vi "SimpleSerialTest.vi"() -> ()   [LabVIEW 2013]
uses:
  Data/TypeDefs/Notifiers.ctl
  Data/TypeDefs/UTM Location.ctl
  Data/TypeDefs/Sail Set Suggestions.ctl
  Data/TypeDefs/Rudder Set Suggestions.ctl
  Data/TypeDefs/OverrideInformation.ctl
  Data/TypeDefs/OverrideMode.ctl
  Data/TypeDefs/MotorSetup.ctl
  Data/TypeDefs/DynamixelSetupInfo.ctl
  Data/TypeDefs/AirmarStatus.ctl
  Data/TypeDefs/HardwareOnline.ctl
  Data/TypeDefs/DynamixelCycleTracker.ctl
  Data/TypeDefs/RC Input Values.ctl
  Classes/Waypoint/Waypoint.lvclass
  Data/TypeDefs/GPS-Compass Queue Cluster.ctl
  Data/TypeDefs/WindData Queue Cluster.ctl
  <vilib>/Instr/_visa.llb/VISA Configure Serial Port (Instr).vi
panel:
  out "Loop Frequency":dbl(graph)
  out "Loop Frequency (Hz)":dbl
  in  "Cycles per buffer flush":i32=1000
  out "Sentence":string
  in  "stop":bool
  out "While counter":i32
  in  "NotifierReff":T1
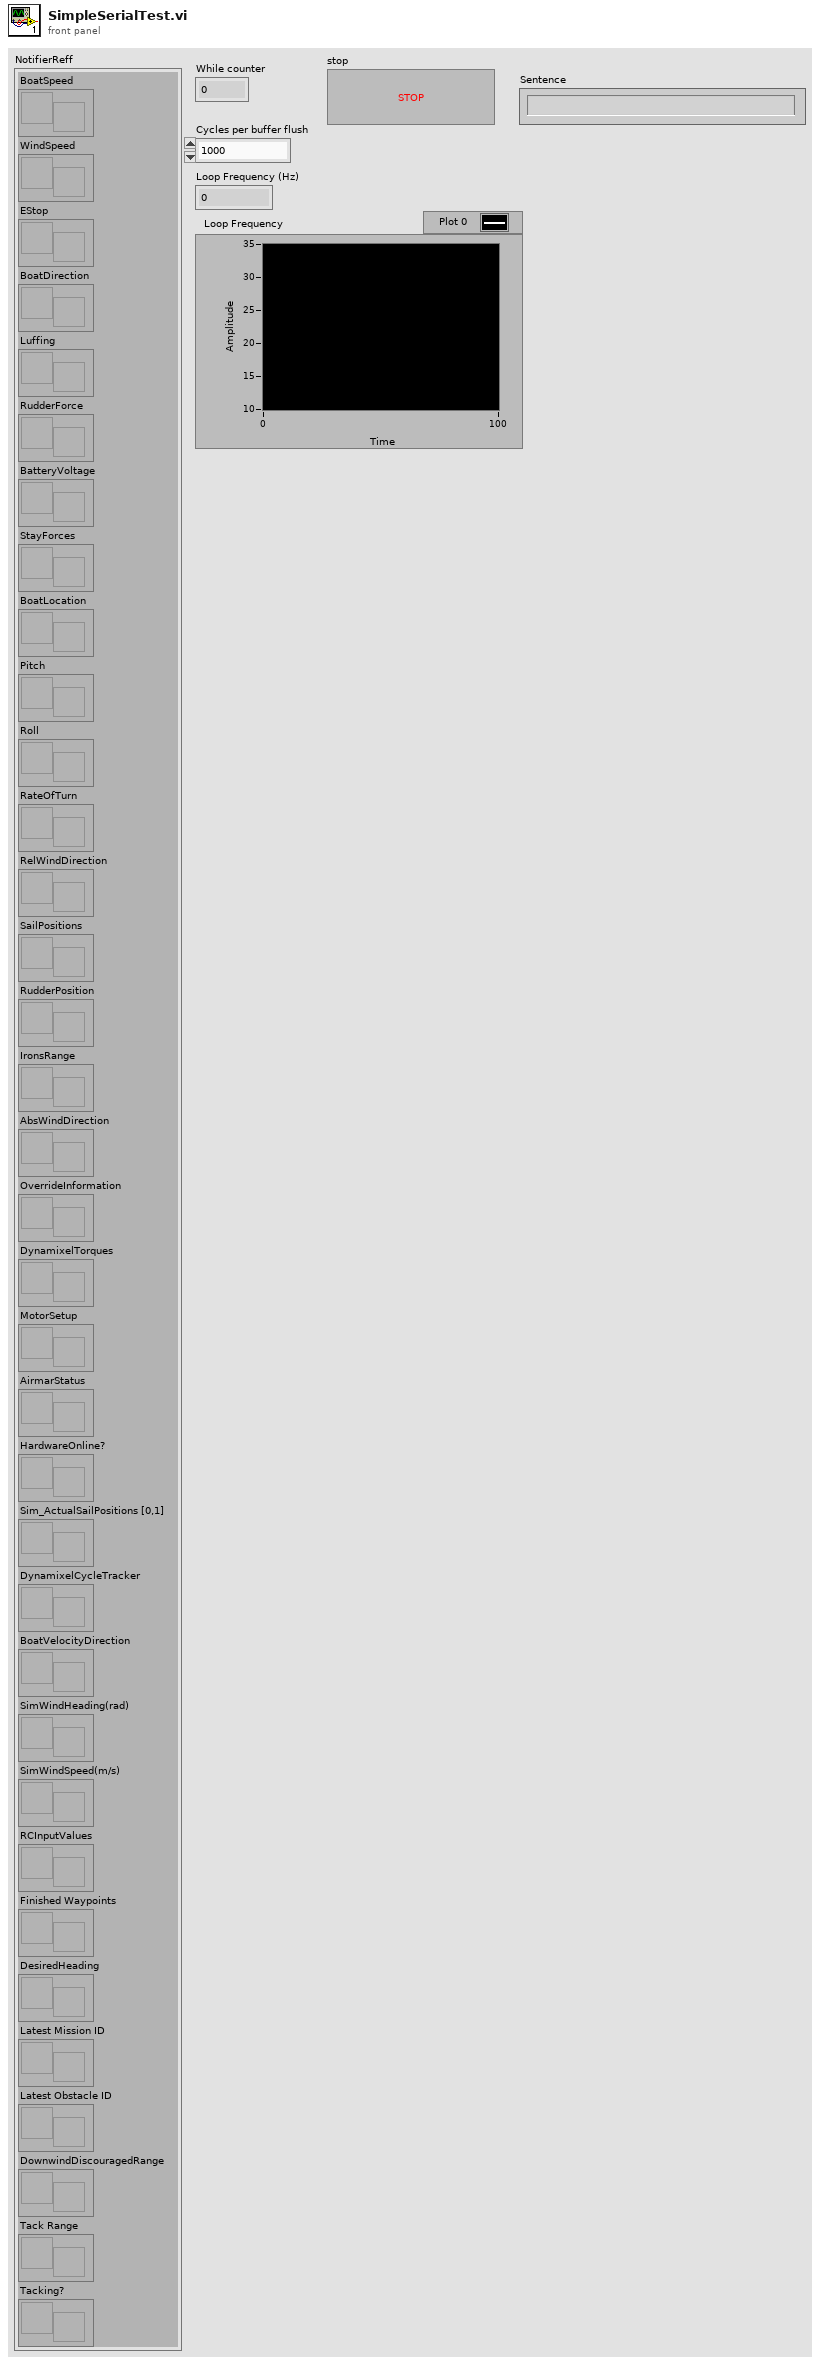
[diagram p1: front panel]
types:
  T1 = typedef "Notifiers.ctl" = cluster{"BoatSpeed":refnum<notifier>, "WindSpeed":refnum<notifier>, "EStop":refnum<notifier>, "BoatDirection":refnum<notifier>, "Luffing":refnum<notifier>, "RudderForce":refnum<notifier>, "BatteryVoltage":refnum<notifier>, "StayForces":refnum<notifier>, "BoatLocation":refnum<notifier>, "Pitch":refnum<notifier>, "Roll":refnum<notifier>, "RateOfTurn":refnum<notifier>, "RelWindDirection":refnum<notifier>, "SailPositions":refnum<notifier>, "RudderPosition":refnum<notifier>, "IronsRange":refnum<notifier>, "AbsWindDirection":refnum<notifier>, "OverrideInformation":refnum<notifier>, "DynamixelTorques":refnum<notifier>, "MotorSetup":refnum<notifier>, "AirmarStatus":refnum<notifier>, "HardwareOnline?":refnum<notifier>, "Sim_ActualSailPositions [0,1]":refnum<notifier>, "DynamixelCycleTracker":refnum<notifier>, "BoatVelocityDirection":refnum<notifier>, "SimWindHeading(rad)":refnum<notifier>, "SimWindSpeed(m/s)":refnum<notifier>, "RCInputValues":refnum<notifier>, "Finished Waypoints":refnum<notifier>, "DesiredHeading":refnum<notifier>, "Latest Mission ID":refnum<notifier>, "Latest Obstacle ID":refnum<notifier>, "DownwindDiscouragedRange":refnum<notifier>, "Tack Range":refnum<notifier>, "Tacking?":refnum<notifier>}
  T2 = typedef "WindData Queue Cluster.ctl" = cluster{"RelWindDirection Queue":refnum<queue>, "WindSpeed Queue":refnum<queue>, "AbsWindDirection Queue":refnum<queue>}
  T3 = typedef "GPS-Compass Queue Cluster.ctl" = cluster{"BoatLocation Queue":refnum<queue>, "BoatDirection Queue":refnum<queue>, "BoatSpeed Queue":refnum<queue>, "RateOfTurn Queue":refnum<queue>, "Pitch Queue":refnum<queue>, "Roll Queue":refnum<queue>, "BoatVelocityDirection Queue ":refnum<queue>}
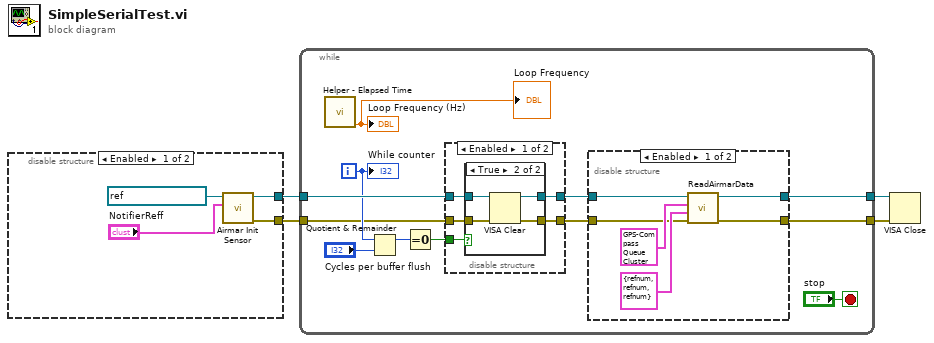
[diagram p0: block diagram]
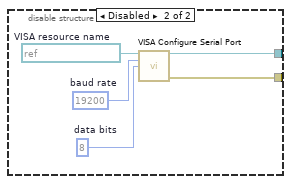
[diagram p2: hidden frame]
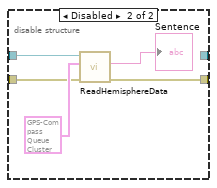
[diagram p5: hidden frame]
diagram:
  n1 = disable-structure shown="Enabled" {
    disable-tunnel: [w6 w10] -> w4
    disable-tunnel: [w5 w9] -> w2
    frame Enabled {
      n2 = call "Airmar Init Sensor.vi"("NotifierReff"="NotifierReff", "VISA Refnum in"=refnum<visa-resource-name> "ASRL2::INSTR") -> ("error out"=w5:errorcluster, "VISA Refnum out"=w6:refnum<visa-resource-name>)  [unwired: 7 in, 1 out]
    }
    frame Disabled {
      w13 = u16 8  # data bits
      w11 = u32 19200  # baud rate
      w12 = refnum<visa-resource-name> "ASRL2::INSTR"  # VISA resource name
      n3 = call-poly "VISA Configure Serial Port"("VISA resource name"=w12, "baud rate (9600)"=w11, "data bits (8)"=w13) -> ("VISA resource name out"=w10:refnum<visa-resource-name>, "error out"=w9:errorcluster)  [unwired: 11 in]
    }
  }
  n4 = while {
    tunnel: w4 -> [w24]
    tunnel: [w18] -> w3
    tunnel: w2 -> [w16]
    tunnel: [w14] -> w1
    i -> [w23]
    stop <- "stop" stop-if-true
    n5 = call "Helper - Elapsed Time.vi"() -> ("Frequency (Hz)"=→"Loop Frequency (Hz)" →"Loop Frequency":dbl)  [unwired: 10 in, 1 out]
    n6 = Quotient & Remainder(x=w23, y="Cycles per buffer flush") -> (x-y*floor(x/y)=w22:i32)  [unwired: 1 out]
    n7 = Equal To 0?(x=w22) -> (x = 0?=w21:bool)
    n8 = disable-structure shown="Enabled" {
      disable-tunnel: [w30 w38] -> w17
      disable-tunnel: w24 -> [w29 w38]
      disable-tunnel: w21 -> [w28 _]
      disable-tunnel: w16 -> [w27 w37]
      disable-tunnel: [w26 w37] -> w15
      frame Enabled {
        n9 = case shown="True" w28 {
          tunnel: [w32 w36] -> w30
          tunnel: w29 -> [w32 w35]
          tunnel: w27 -> [w31 w34]
          tunnel: [w31 w33] -> w26
          frame False {
          }
          frame True {
            n10 = VISA Clear(VISA resource name=w35, error in (no error)=w34) -> (VISA resource name out=w36:refnum<visa-resource-name>, error out=w33:errorcluster)
          }
        }
      }
      frame Disabled {
      }
    }
    n11 = disable-structure shown="Enabled" {
      disable-tunnel: w17 -> [w44 w49]
      disable-tunnel: [w41 _] -> w18
      disable-tunnel: w15 -> [w40 w46]
      disable-tunnel: [w39 w45] -> w14
      frame Enabled {
        n12 = call "ReadAirmarData.vi"("Error in"=w40, "Airmar Wind Queue Cluster"=T2 {"RelWindDirection Queue"=refnum, "WindSpeed Queue"=refnum, "AbsWindDirection Queue"=refnum}, "AirmarGPS-Compass Queue Cluster"=T3 {"BoatLocation Queue"=refnum, "BoatDirection Queue"=refnum, "BoatSpeed Queue"=refnum, "RateOfTurn Queue"=refnum, "Pitch Queue"=refnum, "Roll Queue"=refnum, "BoatVelocityDirection Queue "=refnum}, "VISA UART port"=w44) -> ("Error out"=w39:errorcluster, "VISA UART port Out"=w41:refnum<visa-resource-name>)  [unwired: 5 in, 1 out]
      }
      frame Disabled {
        n13 = call "ReadHemisphereData.vi"("Error in"=w46, "Hemisphere Queue Cluster"=T3 {"BoatLocation Queue"=refnum, "BoatDirection Queue"=refnum, "BoatSpeed Queue"=refnum, "RateOfTurn Queue"=refnum, "Pitch Queue"=refnum, "Roll Queue"=refnum, "BoatVelocityDirection Queue "=refnum}, "VISA UART port"=w49) -> ("Error out"=w45:errorcluster, "Sentence"=→"Sentence":string)  [unwired: 6 in, 1 out]
      }
    }
    "While counter" <- w23
  }
  n14 = VISA Close(VISA resource name=w3, error in (no error)=w1) -> ()  [unwired: 1 out]
